vi "_PC_NS_Wfm_Connect.vi"(8 "error In":errorcluster) -> (0 "error Out":errorcluster, 3 "writer name Out":refnum<k21>)   [LabVIEW 2018]
uses:
  <vilib>/dex/Stream Element Allocation Mode.ctl
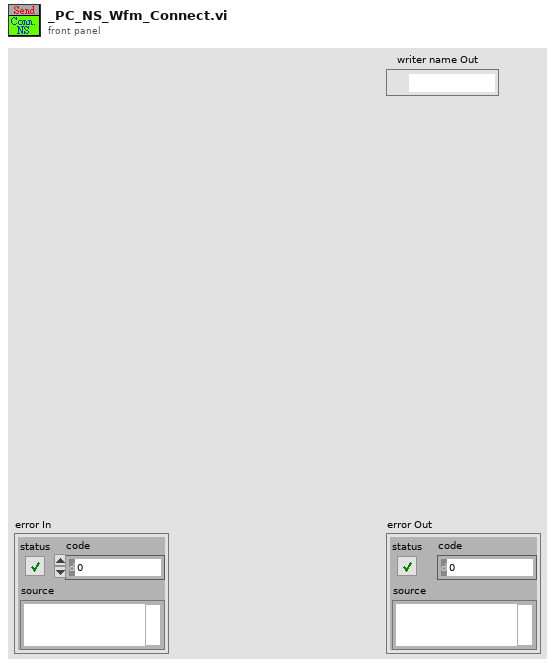
[diagram p1: front panel]
types:
  T1 = typedef "Stream Element Allocation Mode.ctl" = u32
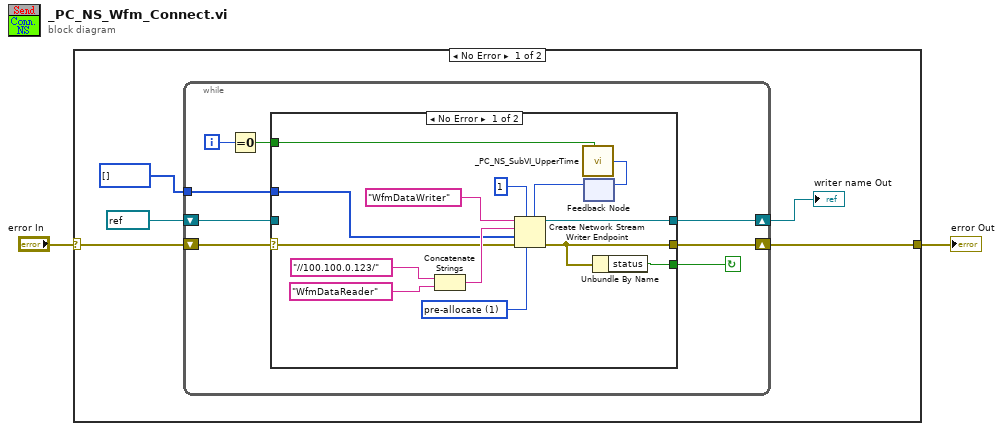
[diagram p0: block diagram]
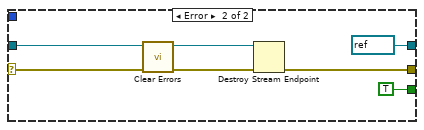
[diagram p2: hidden frame]
diagram:
  n1 = case shown="No Error" "error In" {
    selector: "error In" -> [w3 w36]
    tunnel: [w6 w36] -> w2
    frame No Error {
      n2 = while {
        tunnel: u64[] [] ("WfmData_U64 In") -> [w15]
        shift-right: [w11] -> w6
        shift-left: w3 -> [w14]
        shift-right: [w13] -> w7
        shift-left: refnum<k21> refnum ("writer name") -> [w12]
        i -> [w10]
        stop <- w8 continue-if-true
        n3 = Equal To 0?(x=w10) -> (x = 0?=w9:bool)
        n4 = case shown="No Error" w14 {
          selector: w14 -> [w22 w33]
          tunnel: w15 -> [w23 _]
          tunnel: [w17 w31] -> w11
          tunnel: [w18 refnum<k21> refnum ("writer name")] -> w13
          tunnel: w9 -> [w19 _]
          tunnel: w12 -> [_ w32]
          tunnel: [w16 TRUE] -> w8
          frame No Error {
            w27 = T1 1 items=["allocate as needed", "pre-allocate"] ("element allocation mode")
            n5 = Concatenate Strings("//100.100.0.123/", "WfmDataReader" ("reader url")) -> (w24:string)
            n6 = call "_PC_NS_SubVI_UpperTime.vi"("Init? (F)"=w19) -> ("UpdateTime"=w21:i32)  [unwired: 4 in]
            n7 = feedback-in #1(w21) -> ()
            n8 = feedback #1() -> (w20:i32)  [unwired: 1 in]
            n9 = Create Network Stream Writer Endpoint(5:w20, 6:w27, 7:1 ("writer buffer size"), 8:w22, 9:w23, 10:w24, 11:"WfmDataWriter" ("writer name")) -> (0:w17:errorcluster, 3:w18:refnum<k21>)
            n10 = Unbundle By Name(w17) -> ("status"=w16:bool)
          }
          frame Error {
            n11 = call <vilib>:"Clear Errors.vi"("error in (no error)"=w33) -> ("error out"=w34:errorcluster)  [unwired: 5 in, 1 out]
            n12 = Destroy Stream Endpoint(8:w34, 11:w32) -> (0:w31:errorcluster)
          }
        }
      }
      "writer name Out" <- w7
    }
    frame Error {
    }
  }
  "error Out" <- w2
